vi "Find Param Id match.vi"(10 "RT partial Id in":string, 11 "Id List in":string[](array[string])) -> (1 "found":bool, 2 "Matched id out":string, 3 "Id List out":string[](array[string]))   [LabVIEW 2020, in "Ballard 1553 System Explorer.lvlib"]
uses:
  Ballard 1553 System Explorer.lvlib
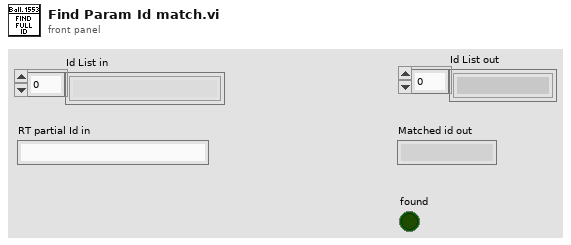
[diagram p1: front panel]
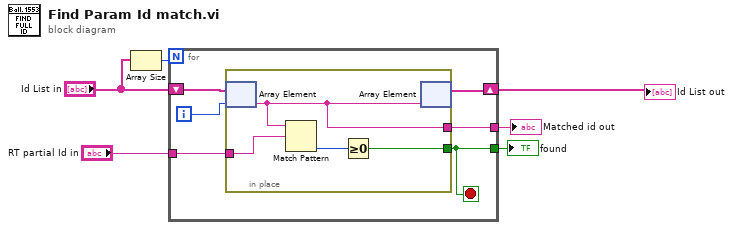
[diagram p0: block diagram]
diagram:
  n1 = Array Size(array="Id List in") -> (size(s)=w2:i32)
  n2 = for {
    N: w2 -> [_]
    shift-right: [w10] -> w6
    shift-left: "Id List in" -> [w12]
    tunnel: "RT partial Id in" -> [w9]
    tunnel: [w8] -> w4
    tunnel: [w7] -> w3
    i -> [w11]
    stop <- w8 stop-if-true
    n3 = in-place {
      in-place-border: w9 -> [w16]
      in-place-border: [w14] -> w8
      in-place-border: [w13] -> w7
      n4 = in-place-array #1(w12, w11) -> (w13:string)
      n5 = Match Pattern(string=w13, regular expression=w16) -> (offset past match=w15:i32)  [unwired: 1 in, 3 out]
      n6 = Greater Or Equal To 0?(x=w15) -> (x >= 0?=w14:bool)
      n7 = in-place-array #1(w13) -> (w10:string[])  [unwired: 1 out]
    }
  }
  "Id List out" <- w6
  "Matched id out" <- w3
  "found" <- w4
